vi "DRC82ReadCtrlPar.vi"(0 "VISA Rsrc":refnum<visa-resource-name>="GPIB0::12::INSTR", 5 "Résistance":u16=25, 11 "error in":errorcluster) -> (4 "Puissance(W)":dbl, 6 "Puissance(%)":i32, 8 "Échelle":u16, 12 "P":u16, 13 "I":u16, 14 "D":u16, 15 "error out":errorcluster)   [LabVIEW 2010]
doc: "Ce Vi interroge l'instrument sur l'échelle de chauffage en watt et le pourcentage de chauffage actuel et retourne une puissance de chauffage en Watts"
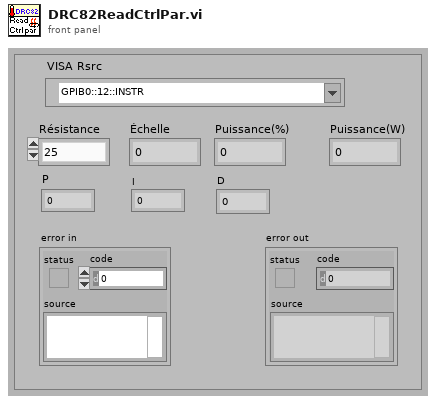
[diagram p1: front panel]
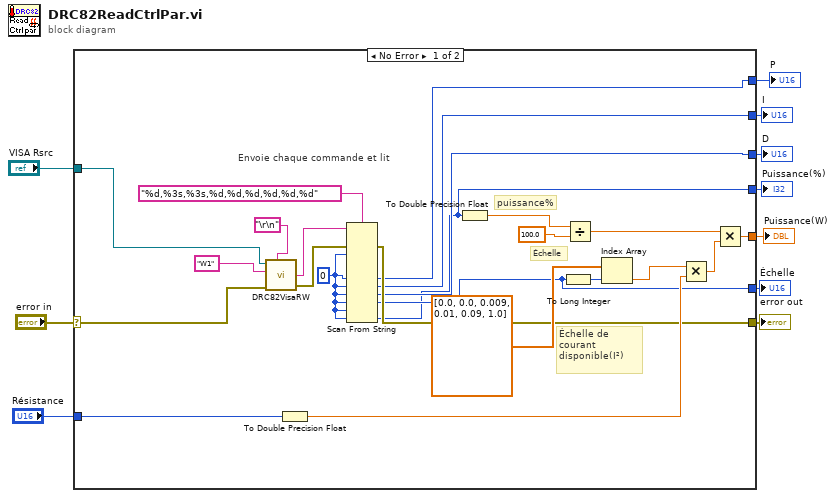
[diagram p0: block diagram]
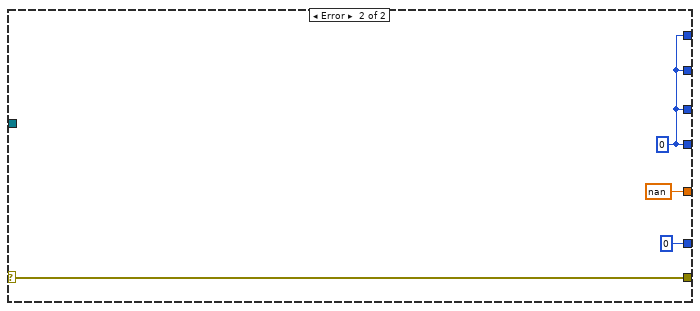
[diagram p2: hidden frame]
diagram:
  n1 = case shown="No Error" "error in" {
    selector: "error in" -> [w33 w38]
    tunnel: [w19 w38] -> w10
    tunnel: "VISA Rsrc" -> [w34 _]
    tunnel: [w31 nan] -> w7
    tunnel: [w12 w35] -> w6
    tunnel: [w13 u16 0] -> w5
    tunnel: "Résistance" -> [w27 _]
    tunnel: [w16 w35] -> w3
    tunnel: [w15 w35] -> w2
    tunnel: [w14 w35] -> w1
    frame No Error {
      w17 = u16 0 ("valeur par défaut 4")
      # "Échelle"
      # "puissance%"
      # "Échelle de courant disponible(I²)"
      # "Envoie chaque commande et lit"
      n2 = call <userlib>:"DRC82VisaRW.vi"("error in (no error)"=w33, "EOS (Aucun)"="\r\n", "ChaineCom"="W1", "VISA Rsrc"=w34) -> ("error out"=w20:errorcluster, "ChaineRep"=w21:string)  [unwired: 3 in, 2 out]
      n3 = To Double Precision Float(number=w27) -> (double precision float=w26:dbl)
      n4 = Scan From String(format string="%d,%3s,%3s,%d,%d,%d,%d,%d,%d" ("chaîne de format"), input string=w21, error in=w20, default 1=w17, default 4=w17, default 5=w17, default 6=w17, default 7=w17, default 8=w17, default 9=w17) -> (error out=w19:errorcluster, output 4=w16:u16, output 5=w15:u16, output 6=w14:u16, output 7=w13:u16, output 9=w12:u16)  [unwired: 7 in, 2 out]
      n5 = To Double Precision Float(number=w12) -> (double precision float=w18:dbl)
      n6 = To Long Integer(number=w13) -> (32bit integer=w29:i32)
      n7 = Divide(x=w18, y=100.0) -> (x/y=w25:dbl)
      n8 = Index Array(array=dbl[] [0.0, 0.0, 0.009, 0.01, 0.09, 1.0], index=w29) -> (element=w28:dbl)
      n9 = Multiply(x=w28, y=w26) -> (x*y=w24:dbl)
      n10 = Multiply(x=w25, y=w24) -> (x*y=w31:dbl)
    }
    frame Error {
      w35 = u16 0
    }
  }
  "error out" <- w10
  "Puissance(W)" <- w7
  "Puissance(%)" <- w6
  "Échelle" <- w5
  "P" <- w3
  "I" <- w2
  "D" <- w1
